vi "Get DataQ Dict.vi"(8 "error in (no error)":errorcluster, 11 "DataQueues in":refnum<class "DataQueues.lvclass">) -> (0 "error out":errorcluster, 2 "DataQ Dict":T1, 3 "DataQueues out":refnum<class "DataQueues.lvclass">)   [LabVIEW 2017, in "DataQueues.lvclass"]
doc: "Developed by Kevin Thompson\nkevin@thompsonengineering.net\n\nCopyright 2018-2020\nThompson Engineering, LLC"
uses:
  DataQueues.lvclass
  <vilib>/TELLC/Dynamic CVT API/TD Dynamic CVT DVR--ref.ctl
  DataQueues.lvclass/DataQueues.ctl
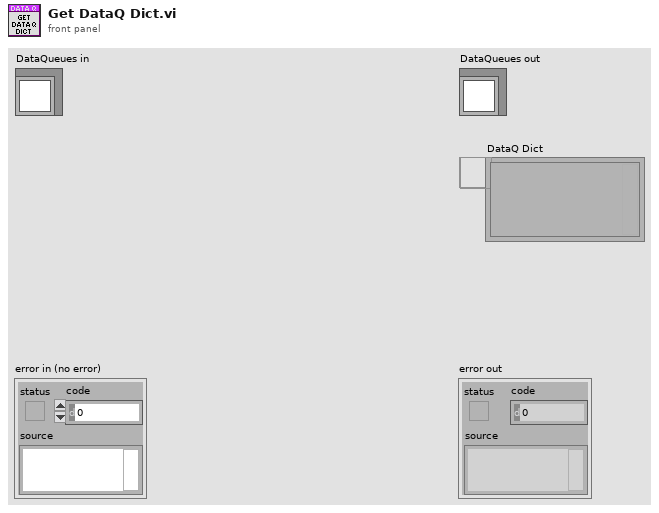
[diagram p1: front panel]
types:
  T1 = typedef "TD Dynamic CVT DVR--ref.ctl" = refnum<data-value>
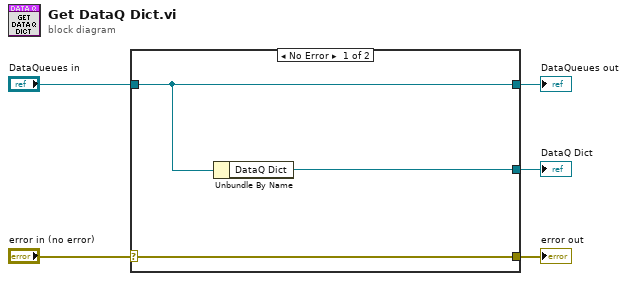
[diagram p0: block diagram]
diagram:
  n1 = case shown="No Error" "error in (no error)" {
    selector: "error in (no error)" -> [w8 w9]
    tunnel: [w8 w9] -> w4
    tunnel: [w7 w10] -> w2
    tunnel: "DataQueues in" -> [w7 w10]
    tunnel: [w6 _] -> w1
    frame No Error {
      n2 = Unbundle By Name(w7) -> ("DataQ Dict"=w6:T1)
    }
    frame Error {
    }
  }
  "error out" <- w4
  "DataQueues out" <- w2
  "DataQ Dict" <- w1
